vi "DMM Switch Handshaking - Cycle Time - Debug.vi"(8 "error in":errorcluster, 11 "file path (use dialog)":path=path "C:/OCVtestfile_debug.json") -> (0 "error out":errorcluster, 2 "Results":T2={"V ch0 Array"=[2.6402355104591723e-06, 3.2050422226470716e-06, 3.2738385547093894e-06, 3.0004056082675545e-06, 3.190429018678622e-06, 3.265655292871135e-06, 3.4283206777974678e-06], "V ch1 Array"=[3.579181433209794e-06, 3.538102305000126e-06, 3.3674070559982216e-06, 3.2951997357567907e-06, 3.0614196043446336e-06, 3.247982674682344e-06, 3.4582756481500834e-06], "V ch2 Array"=[2.636942617106564e-06, 2.444215695573972e-06, 2.3600385872845126e-06, 2.3785120159418297e-06, 2.39158079459529e-06, 2.5415574149365358e-06, 2.629696833600491e-06], "V ch3 Array"=[4.29015971742814e-06, 4.582682915243894e-06, 4.199947801068903e-06, 4.210565880465411e-06, 4.1249236933492e-06, 4.3283146693326225e-06], "V ch4 Array"=[3.2068632920738282e-06, 3.2352868353418705e-06, 3.218523090660476e-06, 3.1985005992771743e-06, 3.2252632419667723e-06, 3.3472279144313767e-06], "Elapsed Time (ms)"=11164, "DMM Fault Array"=[]})   [LabVIEW 2019]
uses:
  OCVResults.ctl
  <instrlib>/niDMM/nidmm.llb/niDMM Acquisition State.ctl
  OCVJSONCluster_debug.ctl
  <instrlib>/niDMM/nidmm.llb/niDMM Measurement Complete.ctl
  <instrlib>/niDMM/nidmm.llb/niDMM Trigger.ctl
  <instrlib>/niDMM/nidmm.llb/niDMM Sample Trigger.ctl
  <instrlib>/niDMM/nidmm.llb/niDMM Configure Measurement Absolute.vi
panel:
  out "SwitchResourceName":string
  out "Backlog":i32
  out "Acq State":T1 caption="Acquisition State"
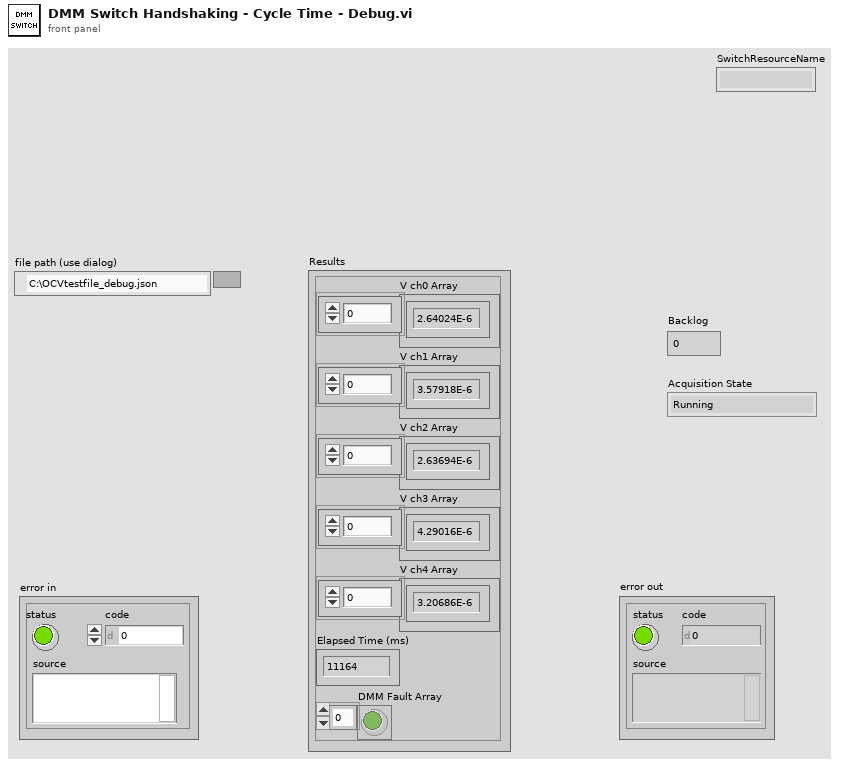
[diagram p1: front panel]
types:
  T1 = typedef "niDMM Acquisition State.ctl" = enum16{"Running", "Finished with Backlog", "Finished with no Backlog", "Paused", "No acquisition in progress"}
  T2 = typedef "OCVResults.ctl" = cluster{"V ch0 Array":dbl[], "V ch1 Array":dbl[], "V ch2 Array":dbl[], "V ch3 Array":dbl[], "V ch4 Array":dbl[], "Elapsed Time (ms)":u32, "DMM Fault Array":bool[]}
  T3 = typedef "niDMM Sample Trigger.ctl" = enum16{"Immediate", "External", "TTL 0", "TTL 1", "TTL 2", "TTL 3", "TTL 4", "TTL 5", "TTL 6", "Interval", "Software", "TTL 7", "PXI Star", "LBR Trig 1", "Aux Trig 1"}
  T4 = typedef "niDMM Trigger.ctl" = enum16{"Immediate", "External", "TTL 0", "TTL 1", "TTL 2", "TTL 3", "TTL 4", "TTL 5", "TTL 6", "Software", "TTL 7", "PXI Star", "LBR Trig 1", "Aux Trig 1"}
  T5 = typedef "niDMM Measurement Complete.ctl" = enum16{"None", "External", "TTL 0", "TTL 1", "TTL 2", "TTL 3", "TTL 4", "TTL 5", "TTL 6", "TTL 7", "LBR Trig 0"}
  T6 = typedef "OCVJSONCluster_debug.ctl" = cluster{"SwitchResourceName":string, "SwitchTopology":string, "SwitchInputTrigger_SoftwareTrigger":i32, "SwitchScanAdvancedOutput_None":i32, "SwitchScanList":string, "DMMResourceName":string, "DMMFunction_DCVolts":i32, "DMMResolution":dbl, "DMMRange":dbl, "DMMTriggerSource_TTL1":i32, "DMMTriggerSlope_RisingEdge":i32, "DMMSampleTrigger_TTL1":i32, "DMMSampleCount":i32, "DMMSampleTriggerSlope_RisingEdge":i32, "DMMMeasurementCompleteTrigger_TTL0":i32, "DMMMeasurementCompleteTriggerSlope_RisingEdge":i32, "DMMApertureTimeUnits_Seconds":i32, "DMMApertureTime":dbl, "DMMNumberOfAverages":i32, "DMMAutoZero_Off":i32, "DMMADCCalibration_Off":i32, "DMMSettleTime":dbl, "DMMControlAction_Commit":i32, "ApplicationLoopCount":i32, "ApplicationNumberOfBatteryCells":i32}
  T7 = enum16{"open", "replace", "create", "open or create", "replace or create", "replace or create with confirmation"}
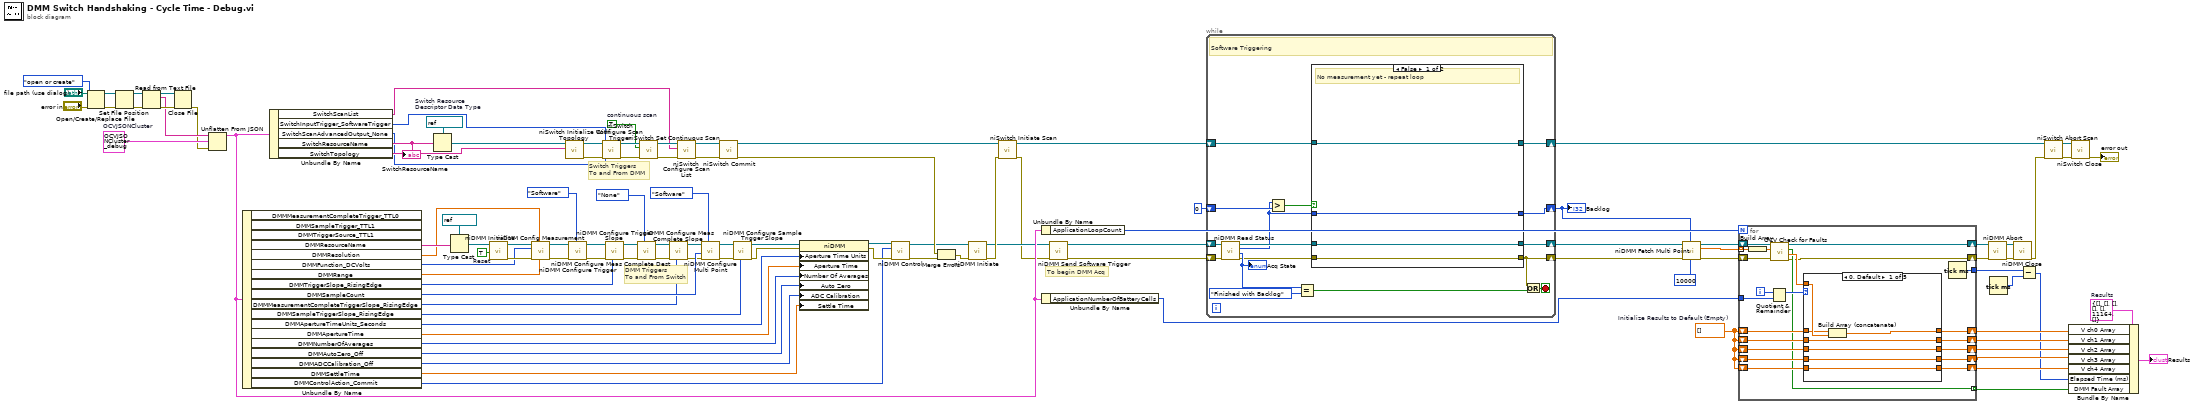
[diagram p0: block diagram]
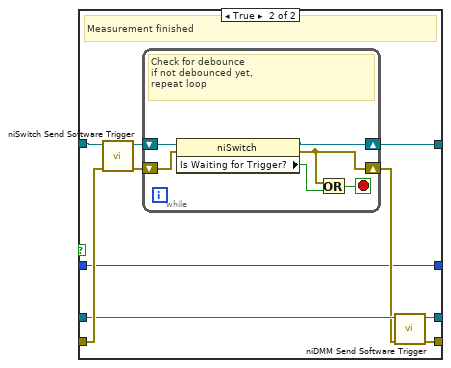
[diagram p2: hidden frame]
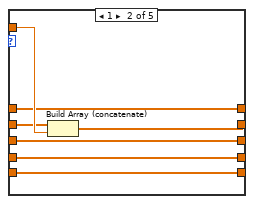
[diagram p3: hidden frame]
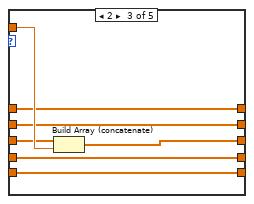
[diagram p4: hidden frame]
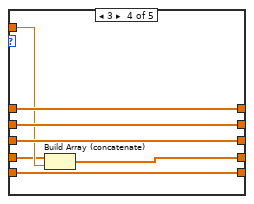
[diagram p5: hidden frame]
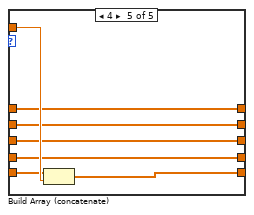
[diagram p6: hidden frame]
diagram:
  w51 = refnum<k15> "Switch"  # Switch Resource Descriptor Data Type
  w73 = T6 {"SwitchResourceName"="", "SwitchTopology"="", "SwitchInputTrigger_SoftwareTrigger"=0, "SwitchScanAdvancedOutput_None"=0, "SwitchScanList"="", "DMMResourceName"="", "DMMFunction_DCVolts"=0, "DMMResolution"=0.0, "DMMRange"=0.0, "DMMTriggerSource_TTL1"=0, "DMMTriggerSlope_RisingEdge"=0, "DMMSampleTrigger_TTL1"=0, "DMMSampleCount"=0, "DMMSampleTriggerSlope_RisingEdge"=0, "DMMMeasurementCompleteTrigger_TTL0"=0, "DMMMeasurementCompleteTriggerSlope_RisingEdge"=0, "DMMApertureTimeUnits_Seconds"=0, "DMMApertureTime"=0.0, "DMMNumberOfAverages"=0, "DMMAutoZero_Off"=0, "DMMADCCalibration_Off"=0, "DMMSettleTime"=0.0, "DMMControlAction_Commit"=0, "ApplicationLoopCount"=0, "ApplicationNumberOfBatteryCells"=0}  # OCVJSONCluster
  w59 = T2 {"V ch0 Array"=[], "V ch1 Array"=[], "V ch2 Array"=[], "V ch3 Array"=[], "V ch4 Array"=[], "Elapsed Time (ms)"=11164, "DMM Fault Array"=[]}  # Results
  w61 = dbl[] []  # Initialize Results to Default (Empty)
  w94 = TRUE  # Reset
  w106 = TRUE  # continuous scan
  # "To begin DMM Acq"
  # "Switch Triggers\nTo and From DMM"
  # "DMM Triggers\nTo and From Switch"
  n1 = Open/Create/Replace File(file path (use dialog)="file path (use dialog)", error in="error in", operation (0:open)=T7."open or create") -> (refnum out=w66:refnum<file>, error out=w65:errorcluster)  [unwired: 3 in, 1 out]
  n2 = Set File Position(refnum=w66, error in=w65) -> (refnum out=w68:refnum<file>, error out=w67:errorcluster)  [unwired: 2 in]
  n3 = Read from Text File(file (use dialog)=w68, error in=w67) -> (refnum out=w70:refnum<file>, text=w64:string, error out=w69:errorcluster)  [unwired: 2 in, 1 out]
  n4 = Close File(refnum=w70, error in=w69) -> (error out=w63:errorcluster)  [unwired: 1 out]
  n5 = Unflatten From JSON(JSON string=w64, type and defaults=w73, error in (no error)=w63) -> (value=w39:T6)  [unwired: 4 in, 1 out]
  n6 = Unbundle By Name(w39) -> ("DMMResourceName"=w38:string, "DMMResolution"=w37:dbl, "DMMFunction_DCVolts"=w43:i32, "DMMRange"=w45:dbl, "DMMTriggerSlope_RisingEdge"=w44:i32, "DMMSampleCount"=w42:i32, "DMMMeasurementCompleteTriggerSlope_RisingEdge"=w20:i32, "DMMSampleTriggerSlope_RisingEdge"=w41:i32, "DMMApertureTimeUnits_Seconds"=w27:i32, "DMMApertureTime"=w26:dbl, "DMMNumberOfAverages"=w25:i32, "DMMAutoZero_Off"=w24:i32, "DMMADCCalibration_Off"=w23:i32, "DMMSettleTime"=w22:dbl, "DMMControlAction_Commit"=w21:i32)  [unwired: 3 out]
  n7 = Unbundle By Name(w39) -> ("SwitchScanList"=w36:string, "SwitchInputTrigger_SoftwareTrigger"=w9:i32, "SwitchScanAdvancedOutput_None"=w8:i32, "SwitchResourceName"=w49:string, "SwitchTopology"=w48:string)
  "SwitchResourceName" <- w49
  n8 = Type Cast(type=w51, x=w49) -> (*(type *) &x=w50:refnum<k15>)
  n9 = Type Cast(type=refnum<k15> "DMM" ("Device Name"), x=w38) -> (*(type *) &x=w46:refnum<k15>)
  n10 = call <instrlib>:"niDMM Initialize.vi"("Reset"=w94, "Instrument Descriptor"=w46) -> ("error out"=w85:errorcluster, "instrument handle out"=w84:refnum<k15>)  [unwired: 8 in]
  n11 = call-poly <instrlib>:"niDMM Config Measurement.vi"("Range"=w45, "Resolution"=w37, "error in (no error)"=w85, "Function"=w43, "instrument handle"=w84) -> ("error out"=w89:errorcluster, "instrument handle out"=w88:refnum<k15>)  [unwired: 5 in]
  n12 = call <instrlib>:"niSwitch Initialize With Topology.vi"("topology name"=w48, "resource name"=w50) -> ("error out"=w103:errorcluster, "instrument handle out"=w104:refnum<k15>)  [unwired: 3 in, 5 out]
  n13 = call <instrlib>:"niDMM Configure Trigger.vi"("Trigger Source"=niDMM_Trigger."Software", "error in (no error)"=w89, "instrument handle"=w88) -> ("error out"=w91:errorcluster, "instrument handle out"=w90:refnum<k15>)  [unwired: 7 in]
  n14 = call <instrlib>:"niSwitch Configure Scan Trigger.vi"("error in (no error)"=w103, "scan advanced output (External)"=w8, "trigger input (External)"=w9, "instrument handle"=w104) -> ("error out"=w107:errorcluster, "instrument handle out"=w109:refnum<k15>)  [unwired: 1 in, 5 out]
  n15 = call <instrlib>:"niDMM Configure Trigger Slope.vi"("Slope"=w44, "error in (no error)"=w91, "instrument handle"=w90) -> ("error out"=w32:errorcluster, "instrument handle out"=w33:refnum<k15>)  [unwired: 7 in]
  n16 = call <instrlib>:"niDMM Configure Meas Complete Dest.vi"("Measurement Complete Destination"=niDMM_Measurement_Complete."None", "error in (no error)"=w32, "instrument handle"=w33) -> ("error out"=w30:errorcluster, "instrument handle out"=w31:refnum<k15>)  [unwired: 7 in]
  n17 = call <instrlib>:"niSwitch Set Continuous Scan.vi"("error in (no error)"=w107, "continuous scan (False)"=w106, "instrument handle"=w109) -> ("error out"=w101:errorcluster, "instrument handle out"=w102:refnum<k15>)  [unwired: 7 out]
  n18 = call <instrlib>:"niDMM Configure Meas Complete Slope.vi"("Slope"=w20, "error in (no error)"=w30, "instrument handle"=w31) -> ("error out"=w29:errorcluster, "instrument handle out"=w28:refnum<k15>)  [unwired: 7 in]
  n19 = call <instrlib>:"niSwitch Configure Scan List.vi"("error in (no error)"=w101, "scan list"=w36, "instrument handle"=w102) -> ("error out"=w100:errorcluster, "instrument handle out"=w99:refnum<k15>)  [unwired: 1 in, 6 out]
  n20 = call <instrlib>:"niDMM Configure Multi Point.vi"("Sample Trigger"=niDMM_Sample_Trigger."Software", "error in (no error)"=w29, "Sample Count"=w42, "instrument handle"=w28) -> ("error out"=w93:errorcluster, "instrument handle out"=w92:refnum<k15>)  [unwired: 6 in]
  n21 = call <instrlib>:"niSwitch Commit.vi"("error in (no error)"=w100, "instrument handle"=w99) -> ("error out"=w83:errorcluster, "instrument handle out"=w98:refnum<k15>)  [unwired: 8 out]
  n22 = call <instrlib>:"niDMM Configure Sample Trigger Slope.vi"("Slope"=w41, "error in (no error)"=w93, "instrument handle"=w92) -> ("error out"=w78:errorcluster, "instrument handle out"=w79:refnum<k15>)  [unwired: 7 in]
  n23 = property class="niDMM"(reference=w79, error in=w78, "Aperture Time Units"=w27, "Aperture Time"=w26, "Number Of Averages"=w25, "Auto Zero"=w24, "ADC Calibration"=w23, "Settle Time"=w22) -> (reference out=w75:refnum<k15>, error out=w74:errorcluster)
  n24 = call <instrlib>:"niDMM Control.vi"("error in (no error)"=w74, "Control Action"=w21, "instrument handle"=w75) -> ("error out"=w82:errorcluster, "instrument handle out"=w80:refnum<k15>)  [unwired: 7 in]
  n25 = Merge Errors(w83, w82) -> (w81:errorcluster)
  n26 = call <instrlib>:"niDMM Initiate.vi"("error in (no error)"=w81, "instrument handle"=w80) -> ("error out"=w35:errorcluster, "instrument handle out"=w13:refnum<k15>)  [unwired: 8 in]
  n27 = call <instrlib>:"niSwitch Initiate Scan.vi"("error in (no error)"=w35, "instrument handle"=w98) -> ("error out"=w12:errorcluster, "instrument handle out"=w11:refnum<k15>)  [unwired: 8 out]
  n28 = Unbundle By Name(w39) -> ("ApplicationLoopCount"=w19:i32)
  n29 = Unbundle By Name(w39) -> ("ApplicationNumberOfBatteryCells"=w40:i32)
  n30 = call <instrlib>:"niDMM Send Software Trigger.vi"("error in (no error)"=w12, "instrument handle"=w13) -> ("error out"=w3:errorcluster, "instrument handle out"=w4:refnum<k15>)  [unwired: 8 in]
  n31 = while {
    shift-right: [w117] -> w2
    shift-left: w4 -> [w125]
    shift-right: [w110] -> w1
    shift-left: w3 -> [w124]
    shift-right: [w112] -> w10
    shift-left: 0 ("Backlog") -> [w120]
    shift-right: [w118] -> _
    shift-left: w11 -> [w121]
    stop <- w115 stop-if-true
    # "Software Triggering"
    n32 = call <instrlib>:"niDMM Read Status.vi"("error in (no error)"=w124, "instrument handle"=w125) -> ("error out"=w111:errorcluster, "Acquisition State"=w123:T1, "Backlog"=w113:i32, "instrument handle out"=w116:refnum<k15>)  [unwired: 6 in]
    "Acq State" <- w123
    n33 = Greater?(x=w113, y=w120) -> (0:w119:bool)
    n34 = Equal?(x=w123, y=niDMM_Acquisition_State."Finished with Backlog") -> (x = y?=w114:bool)
    n35 = case shown="False" w119 {
      tunnel: w121 -> [w129 w139]
      tunnel: w111 -> [w126 w136]
      tunnel: [w129 w135] -> w118
      tunnel: [w127 w134] -> w117
      tunnel: [w126 w133] -> w110
      tunnel: w116 -> [w127 w132]
      tunnel: w113 -> [w128 w130]
      tunnel: [w128 w130] -> w112
      frame False {
        # "No measurement yet - repeat loop"
      }
      frame True {
        # "Measurement finished"
        n36 = call <instrlib>:"niSwitch Send Software Trigger.vi"("error in (no error)"=w136, "instrument handle"=w139) -> ("error out"=w137:errorcluster, "instrument handle out"=w138:refnum<k15>)  [unwired: 8 in]
        n37 = while {
          shift-right: [w143] -> w135
          shift-left: w138 -> [w145]
          shift-right: [w140] -> w131
          shift-left: w137 -> [w144]
          stop <- w141 stop-if-true
          # "Check for debounce\nif not debounced yet, \nrepeat loop"
          n38 = property class="niSwitch"(reference=w145, error in=w144) -> (reference out=w143:refnum<k15>, error out=w140:errorcluster, "Is Waiting for Trigger?"=w142:bool)
          n39 = Or(x=w140, y=w142) -> (x .or. y?=w141:bool)
        }
        n40 = call <instrlib>:"niDMM Send Software Trigger.vi"("error in (no error)"=w131, "instrument handle"=w132) -> ("error out"=w133:errorcluster, "instrument handle out"=w134:refnum<k15>)  [unwired: 8 in]
      }
    }
    n41 = Or(x=w110, y=w114) -> (x .or. y?=w115:bool)
  }
  "Backlog" <- w10
  n42 = call <instrlib>:"niDMM Fetch Multi Point.vi"("Maximum Time (msec)"=10000, "Number to Fetch"=w10, "error in (no error)"=w1, "instrument handle"=w2) -> ("error out"=w18:errorcluster, "Measurements"=w15:dbl[], "instrument handle out"=w17:refnum<k15>)  [unwired: 4 in, 1 out]
  n43 = for {
    N: w19 -> [_]
    shift-right: [w150] -> w77
    shift-left: w18 -> [w149]
    tunnel: [w166] -> w96
    shift-right: [w147] -> w76
    shift-left: w17 -> [w147]
    shift-right: [w163] -> w60
    shift-left: w61 -> [w162]
    shift-right: [w161] -> w55
    shift-left: w61 -> [w160]
    shift-right: [w159] -> w56
    shift-left: w61 -> [w158]
    shift-right: [w157] -> w57
    shift-left: w61 -> [w156]
    shift-right: [w155] -> w58
    shift-left: w61 -> [w154]
    tunnel: [w152] -> w52 mode=indexing
    tunnel: w40 -> [w151]
    tunnel: w15 -> [w146] mode=indexing
    i -> [w165]
    n44 = Build Array(w146) -> (w148:dbl[])
    n45 = call "OCV Check for Faults.vi"("Error In"=w149, "dmm voltage measurements"=w148) -> ("Error Out"=w150:errorcluster, "Voltage Out"=w153:dbl, "DMM Fault"=w152:bool)  [unwired: 7 in]
    n46 = Quotient & Remainder(x=w165, y=w151) -> (x-y*floor(x/y)=w164:i32)  [unwired: 1 out]
    n47 = case shown="0, Default" w164 {
      tunnel: w153 -> [w173 w180 w187 w191 w201]
      tunnel: [w172 w177 w184 w194 w198] -> w163
      tunnel: w162 -> [w171 w177 w184 w194 w198]
      tunnel: [w170 w179 w183 w193 w197] -> w161
      tunnel: w160 -> [w170 w178 w183 w193 w197]
      tunnel: [w169 w176 w186 w192 w196] -> w159
      tunnel: w158 -> [w169 w176 w185 w192 w196]
      tunnel: [w168 w175 w182 w190 w195] -> w157
      tunnel: w156 -> [w168 w175 w182 w189 w195]
      tunnel: [w167 w174 w181 w188 w200] -> w155
      tunnel: w154 -> [w167 w174 w181 w188 w199]
      frame 0, Default {
        n48 = Build Array (concatenate)(w171, w173) -> (w172:dbl[])
      }
      frame 1 {
        n49 = Build Array (concatenate)(w178, w180) -> (w179:dbl[])
      }
      frame 2 {
        n50 = Build Array (concatenate)(w185, w187) -> (w186:dbl[])
      }
      frame 3 {
        n51 = Build Array (concatenate)(w189, w191) -> (w190:dbl[])
      }
      frame 4 {
        n52 = Build Array (concatenate)(w199, w201) -> (w200:dbl[])
      }
    }
    n53 = Tick Count (ms)() -> (millisecond timer value=w166:u32)
  }
  n54 = call <instrlib>:"niDMM Abort.vi"("error in (no error)"=w77, "instrument handle"=w76) -> ("error out"=w87:errorcluster, "instrument handle out"=w86:refnum<k15>)  [unwired: 8 in]
  n55 = Tick Count (ms)() -> (millisecond timer value=w95:u32)
  n56 = call <instrlib>:"niDMM Close.vi"("error in (no error)"=w87, "instrument handle"=w86) -> ("error out"=w34:errorcluster)  [unwired: 9 in]
  n57 = Subtract(x=w96, y=w95) -> (x-y=w53:u32)
  n58 = call <instrlib>:"niSwitch Abort Scan.vi"("error in (no error)"=w34, "instrument handle"=w11) -> ("error out"=w105:errorcluster, "instrument handle out"=w108:refnum<k15>)  [unwired: 8 out]
  n59 = Bundle By Name(cluster=w59, "V ch0 Array"=w60, "V ch1 Array"=w55, "V ch2 Array"=w56, "V ch3 Array"=w57, "V ch4 Array"=w58, "Elapsed Time (ms)"=w53, "DMM Fault Array"=w52) -> (→"Results":T2)
  n60 = call <instrlib>:"niSwitch Close.vi"("error in (no error)"=w105, "instrument handle"=w108) -> ("error out"=→"error out":errorcluster)  [unwired: 9 out]
